vi "GuardaCorreccions.vi"(9 "CorreccioPos":T1, 10 "CorreccioNeg":T1, 11 "String":string) -> ()   [LabVIEW 2017]
uses:
  <vilib>/registry/registry.llb/Registry RtKey.ctl
  <vilib>/registry/registry.llb/Write Registry Value Simple STR.vi
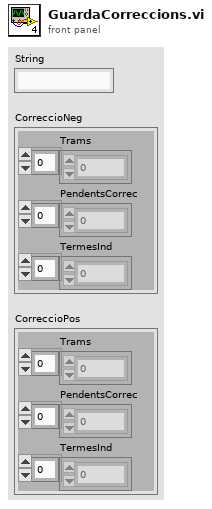
[diagram p1: front panel]
types:
  T1 = cluster{"Trams":dbl[], "PendentsCorrec":dbl[], "TermesInd":dbl[]}
  T2 = typedef "Registry RtKey.ctl" = enum32{"HKEY_CLASSES_ROOT", "HKEY_CURRENT_USER", "HKEY_LOCAL_MACHINE", "HKEY_USERS", "HKEY_PERFORMANCE_DATA", "HKEY_CURRENT_CONFIG", "HKEY_DYN_DATA"}
  T3 = typedef "Registry refnum.ctl" = refnum<k1>
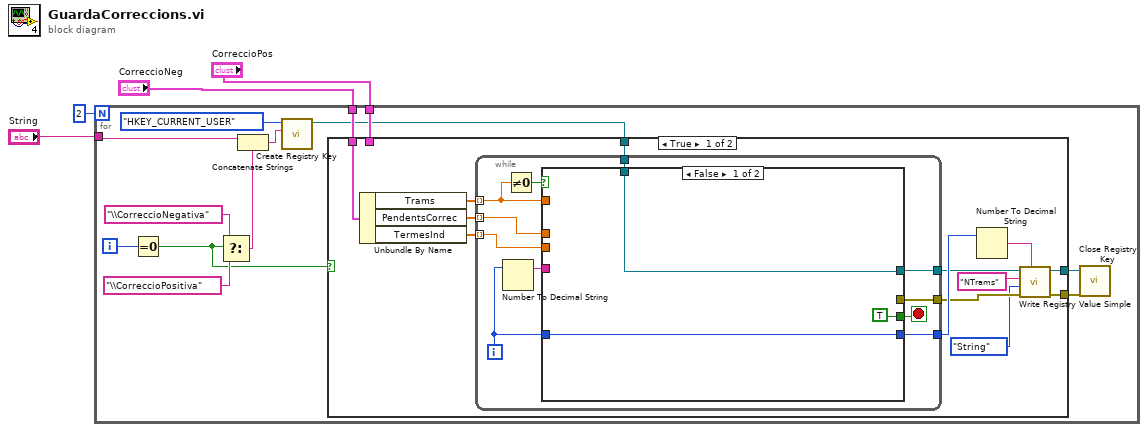
[diagram p0: block diagram]
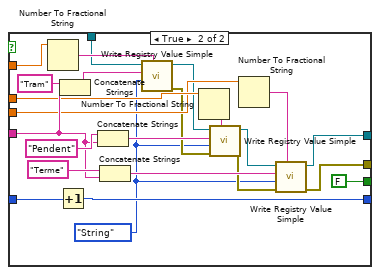
[diagram p2: hidden frame]
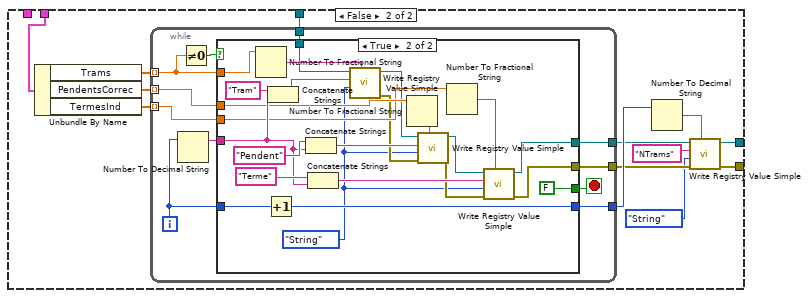
[diagram p3: hidden frame]
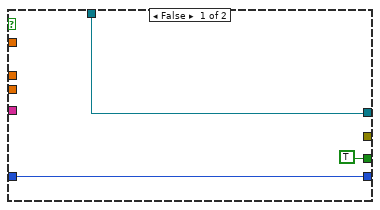
[diagram p4: hidden frame]
diagram:
  n1 = for {
    N: 2 -> [_]
    tunnel: "CorreccioPos" -> [w10]
    tunnel: "CorreccioNeg" -> [w11]
    tunnel: "String" -> [w14]
    i -> [w15]
    n2 = Equal To 0?(x=w15) -> (x = 0?=w12:bool)
    n3 = Select(t="\\CorreccioNegativa" ("subkey"), s=w12, f="\\CorreccioPositiva" ("subkey")) -> (s? t:f=w13:string)
    n4 = Concatenate Strings(w14, w13) -> (w5:string)
    n5 = call <vilib>:"Create Registry Key.vi"("subkey"=w5, "root key (HKEY_LOCAL_MACHINE)"=Registry_RtKey."HKEY_CURRENT_USER") -> ("refnum out"=w7:T3)  [unwired: 7 in, 2 out]
    n6 = case shown="True" w12 {
      tunnel: w11 -> [w19 _]
      tunnel: w10 -> [_ w69]
      tunnel: w7 -> [w27 w78]
      tunnel: [w22 w73] -> w9
      tunnel: [w21 w72] -> w8
      frame True {
        n7 = Unbundle By Name(w19) -> ("Trams"=w30:dbl[], "PendentsCorrec"=w29:dbl[], "TermesInd"=w28:dbl[])
        n8 = while {
          tunnel: w30 -> [w33] mode=indexing
          tunnel: w29 -> [w38] mode=indexing
          tunnel: w28 -> [w37] mode=indexing
          tunnel: w27 -> [w36]
          tunnel: [w31] -> w26
          tunnel: [w35] -> w23
          tunnel: [w34] -> w20
          i -> [w32]
          stop <- w40 stop-if-true
          n9 = Number To Decimal String(number=w32) -> (decimal integer string=w39:string)  [unwired: 1 in]
          n10 = Not Equal To 0?(x=w33) -> (x != 0?=w41:bool)
          n11 = case shown="False" w41 {
            tunnel: [TRUE FALSE] -> w40
            tunnel: w33 -> [_ w67]
            tunnel: w39 -> [_ w60]
            tunnel: w38 -> [_ w56]
            tunnel: w37 -> [_ w55]
            tunnel: w36 -> [w43 w54]
            tunnel: [w43 w49] -> w35
            tunnel: [_ w48] -> w34
            tunnel: w32 -> [w42 w47]
            tunnel: [w42 w46] -> w31
            frame False {
            }
            frame True {
              w45 = enum16{"String", "Binary", "DWORD"}."String" ("simple data type")
              n12 = Number To Fractional String(number=w67) -> (F-format string=w66:string)  [unwired: 3 in]
              n13 = Increment(x=w47) -> (x+1=w46:i32)
              n14 = Concatenate Strings("Tram" ("value"), w60) -> (w64:string)
              n15 = Concatenate Strings("Pendent" ("value"), w60) -> (w62:string)
              n16 = Concatenate Strings("Terme" ("value"), w60) -> (w59:string)
              n17 = call-poly <vilib>:"Write Registry Value Simple.vi"("String/Binary data"=w66, "simple data type"=w45, "value"=w64, "refnum"=w54) -> ("error out"=w50:errorcluster, "refnum out"=w53:T3)  [unwired: 4 in]
              n18 = Number To Fractional String(number=w56) -> (F-format string=w58:string)  [unwired: 3 in]
              n19 = call-poly <vilib>:"Write Registry Value Simple.vi"("String/Binary data"=w58, "error in (no error)"=w50, "simple data type"=w45, "value"=w62, "refnum"=w53) -> ("error out"=w51:errorcluster, "refnum out"=w52:T3)  [unwired: 3 in]
              n20 = Number To Fractional String(number=w55) -> (F-format string=w57:string)  [unwired: 3 in]
              n21 = call-poly <vilib>:"Write Registry Value Simple.vi"("String/Binary data"=w57, "error in (no error)"=w51, "simple data type"=w45, "value"=w59, "refnum"=w52) -> ("error out"=w48:errorcluster, "refnum out"=w49:T3)  [unwired: 3 in]
            }
          }
        }
        n22 = Number To Decimal String(number=w26) -> (decimal integer string=w25:string)  [unwired: 1 in]
        n23 = call-poly <vilib>:"Write Registry Value Simple.vi"("String/Binary data"=w25, "error in (no error)"=w20, "simple data type"=enum16{"String", "Binary", "DWORD"}."String", "value"="NTrams", "refnum"=w23) -> ("error out"=w21:errorcluster, "refnum out"=w22:T3)  [unwired: 3 in]
      }
      frame False {
        n24 = Unbundle By Name(w69) -> ("Trams"=w81:dbl[], "PendentsCorrec"=w80:dbl[], "TermesInd"=w79:dbl[])
        n25 = while {
          tunnel: w81 -> [w84] mode=indexing
          tunnel: w80 -> [w89] mode=indexing
          tunnel: w79 -> [w88] mode=indexing
          tunnel: w78 -> [w87]
          tunnel: [w82] -> w77
          tunnel: [w86] -> w74
          tunnel: [w85] -> w71
          i -> [w83]
          stop <- w91 stop-if-true
          n26 = Number To Decimal String(number=w83) -> (decimal integer string=w90:string)  [unwired: 1 in]
          n27 = Not Equal To 0?(x=w84) -> (x != 0?=w92:bool)
          n28 = case shown="True" w92 {
            tunnel: [TRUE FALSE] -> w91
            tunnel: w84 -> [_ w118]
            tunnel: w90 -> [_ w111]
            tunnel: w89 -> [_ w107]
            tunnel: w88 -> [_ w106]
            tunnel: w87 -> [w94 w105]
            tunnel: [w94 w100] -> w86
            tunnel: [_ w99] -> w85
            tunnel: w83 -> [w93 w98]
            tunnel: [w93 w97] -> w82
            frame False {
            }
            frame True {
              w96 = enum16{"String", "Binary", "DWORD"}."String" ("simple data type")
              n29 = Number To Fractional String(number=w118) -> (F-format string=w117:string)  [unwired: 3 in]
              n30 = Increment(x=w98) -> (x+1=w97:i32)
              n31 = Concatenate Strings("Tram" ("value"), w111) -> (w115:string)
              n32 = Concatenate Strings("Pendent" ("value"), w111) -> (w113:string)
              n33 = Concatenate Strings("Terme" ("value"), w111) -> (w110:string)
              n34 = call-poly <vilib>:"Write Registry Value Simple.vi"("String/Binary data"=w117, "simple data type"=w96, "value"=w115, "refnum"=w105) -> ("error out"=w101:errorcluster, "refnum out"=w104:T3)  [unwired: 4 in]
              n35 = Number To Fractional String(number=w107) -> (F-format string=w109:string)  [unwired: 3 in]
              n36 = call-poly <vilib>:"Write Registry Value Simple.vi"("String/Binary data"=w109, "error in (no error)"=w101, "simple data type"=w96, "value"=w113, "refnum"=w104) -> ("error out"=w102:errorcluster, "refnum out"=w103:T3)  [unwired: 3 in]
              n37 = Number To Fractional String(number=w106) -> (F-format string=w108:string)  [unwired: 3 in]
              n38 = call-poly <vilib>:"Write Registry Value Simple.vi"("String/Binary data"=w108, "error in (no error)"=w102, "simple data type"=w96, "value"=w110, "refnum"=w103) -> ("error out"=w99:errorcluster, "refnum out"=w100:T3)  [unwired: 3 in]
            }
          }
        }
        n39 = Number To Decimal String(number=w77) -> (decimal integer string=w76:string)  [unwired: 1 in]
        n40 = call-poly <vilib>:"Write Registry Value Simple.vi"("String/Binary data"=w76, "error in (no error)"=w71, "simple data type"=enum16{"String", "Binary", "DWORD"}."String", "value"="NTrams", "refnum"=w74) -> ("error out"=w72:errorcluster, "refnum out"=w73:T3)  [unwired: 3 in]
      }
    }
    n41 = call <vilib>:"Close Registry Key.vi"("error in (no error)"=w8, "refnum"=w9) -> ()  [unwired: 5 in, 1 out]
  }
